vi "convert_a_b.vi"(10 "Numeric Arrays":dbl format="%#_13g") -> (2 "Output":dbl)   [LabVIEW 2014]
panel:
  # "Conversion from A - B\n\nThe data for this is not available"
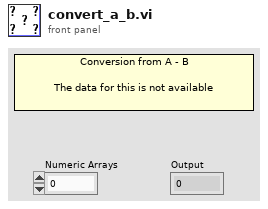
[diagram p1: front panel]
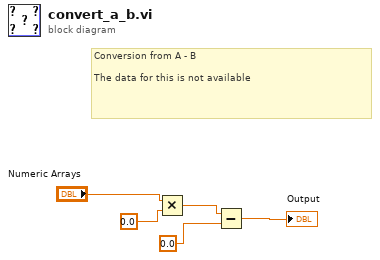
[diagram p0: block diagram]
diagram:
  # "Conversion from A - B\n\nThe data for this is not available"
  n1 = Multiply(x="Numeric Arrays", y=0.0) -> (x*y=w5:dbl)
  n2 = Subtract(x=w5, y=0.0) -> (x-y=→"Output":dbl)
